vi "NI VeriStand - Set Parameter 2D Array Values.vi"(7 "Target":string, 8 "error in (no error)":errorcluster, 9 "Values":dbl[][](array[numeric]), 10 "Parameter":string, 11 "ModelManager in":T1) -> (0 "error out":errorcluster, 3 "ModelManager out":T1)   [LabVIEW 2020, in "NI_VS ModelManager ExecutionAPI.lvlib"]
doc: "Sets values of model parameters present on the target. You must manually select the polymorphic instance to use."
uses:
  <vilib>/NI VeriStand/Execution/ModelManager/NI_VS ModelManager ExecutionAPI.lvlib
  <vilib>/NI VeriStand/Execution/ModelManager/ModelManagerAPI.ctl
  NationalInstruments.VeriStand.ClientAPI
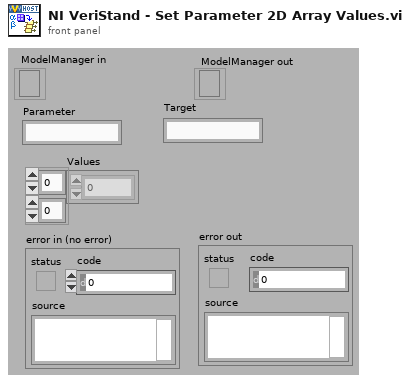
[diagram p1: front panel]
types:
  T1 = typedef "NI_VS ModelManager ExecutionAPI.lvlib/ModelManagerAPI.ctl" = refnum<k24>
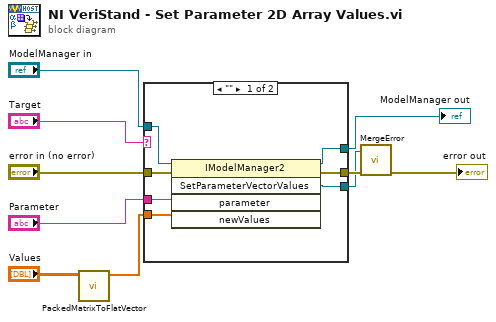
[diagram p0: block diagram]
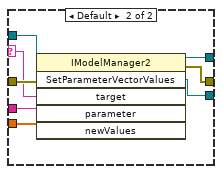
[diagram p2: hidden frame]
diagram:
  n1 = call <vilib>:"PackedMatrixToFlatVector.vi"("Matrix"="Values") -> ("FlatVector"=w2:dbl[])  [unwired: 10 out]
  n2 = case shown="\"\"" "Target" {
    selector: "Target" -> [_ w18]
    tunnel: "ModelManager in" -> [w17 w25]
    tunnel: [w16 w24] -> w9
    tunnel: [w15 w23] -> w8
    tunnel: [w14 w22] -> w7
    tunnel: "error in (no error)" -> [w13 w21]
    tunnel: "Parameter" -> [w12 w20]
    tunnel: w2 -> [w11 w19]
    frame "" {
      n3 = invoke class="IModelManager2" method="SetParameterVectorValues"(reference=w17, error in=w13, "parameter"=w12, "newValues"=w11) -> (reference out=w16:T1, error out=w15:errorcluster, "SetParameterVectorValues"=w14:refnum<k24>)  [unwired: 1 in, 2 out]
    }
    frame Default {
      n4 = invoke class="IModelManager2" method="SetParameterVectorValues"(reference=w25, error in=w21, "target"=w18, "parameter"=w20, "newValues"=w19) -> (reference out=w24:T1, error out=w23:errorcluster, "SetParameterVectorValues"=w22:refnum<k24>)  [unwired: 1 in, 3 out]
    }
  }
  "ModelManager out" <- w9
  n5 = call <vilib>:"MergeError.vi"("error in (no error)"=w8, "Error"=w7) -> ("error out"=→"error out":errorcluster)  [unwired: 9 out]
